vi "T7_I2CRead_UINT16_Register.vi"(9 "FirstChannel":i32, 10 "Remote Port":u16=502, 11 "Remote IP Address":string="192.168.124.53") -> (1 "Raw Data Read":u16[](array[numeric]), 2 "LastValue":dbl, 3 "Array":dbl[](array[numeric]))   [LabVIEW 2014]
uses:
  Serial Link Layer/NI_Modbus_Cleaned/NI Modbus121Clean.llb/MB Ethernet Master Query Read Input Registers (poly).vi
panel:
  in  "Num Registers to read":i32=2
  out "Read UINT16":u16
  # "MB Ethernet Example Master.vi\n\nInstructions\n1.Use Kipling to find your devices IP address & modify the\n\"Remote IP Addres\"\n2. Run this VI\n3. Change value of \"UINT16 to Write\" & press \"Write Data\""
  # "TCP Parameters"
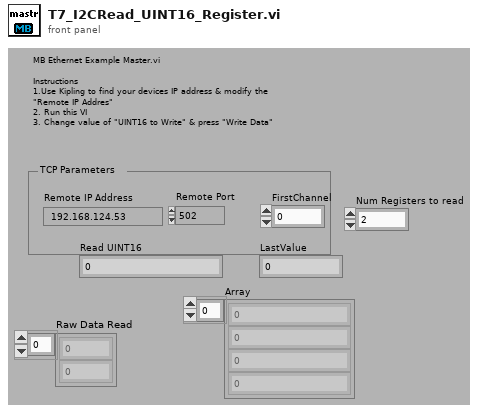
[diagram p1: front panel]
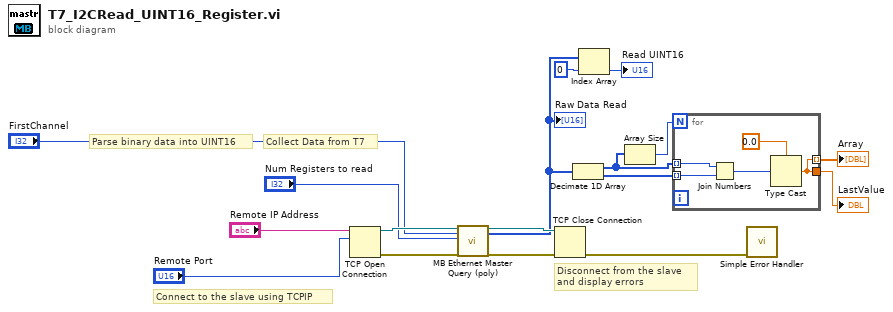
[diagram p0: block diagram]
diagram:
  # "Parse binary data into UINT16"
  # "Collect Data from T7"
  # "Disconnect from the slave\nand display errors"
  # "Connect to the slave using TCPIP"
  n1 = TCP Open Connection(address="Remote IP Address", remote port or service name="Remote Port") -> (connection ID=w15:refnum<k5>, error out=w14:errorcluster)  [unwired: 3 in]
  n2 = call-poly "MB Ethernet Master Query (poly).vi"("TCP Connection Refnum in"=w15, "Starting Address"="FirstChannel", "Quantity"="Num Registers to read", "error in"=w14) -> ("TCP Connection Refnum (dup)"=w11:refnum<k5>, "Input Registers"=w2:u16[], "error out"=w12:errorcluster)  [unwired: 12 in, 1 out]
  "Raw Data Read" <- w2
  n3 = TCP Close Connection(connection ID=w11, error in (no error)=w12) -> (error out=w13:errorcluster)  [unwired: 2 out]
  n4 = Decimate 1D Array(w2) -> (w4:u16[], w5:u16[])
  n5 = Index Array(array=w2, index=0) -> (element=→"Read UINT16":u16)
  n6 = Array Size(array=w4) -> (size(s)=w3:i32)
  n7 = for {
    N: w3 -> [_]
    tunnel: w4 -> [w21] mode=indexing
    tunnel: w5 -> [w22] mode=indexing
    tunnel: [w18] -> w6 mode=indexing
    tunnel: [w18] -> w7
    n8 = Join Numbers(hi=w21, lo=w22) -> ((hi.lo)=w20:u32)
    n9 = Type Cast(type=sgl 0.0, x=w20) -> (*(type *) &x=w18:sgl)
  }
  "Array" <- w6
  "LastValue" <- w7
  n10 = call <vilib>:"Simple Error Handler.vi"("error in (no error)"=w13) -> ()  [unwired: 1 in, 8 out]
